vi "readString.vi"(8 "error in (no error)":errorcluster, 10 "Length":i32, 11 "ModbusBuffer in":refnum<class "ModbusBuffer.lvclass">) -> (0 "error out":errorcluster, 2 "Output":string, 3 "ModbusBuffer out":refnum<class "ModbusBuffer.lvclass">)   [LabVIEW 2016, in "RTModbus.lvlib" / "ModbusBuffer.lvclass"]
uses:
  ModbusBuffer.lvclass
  ModbusBuffer.lvclass/ModbusBuffer.ctl
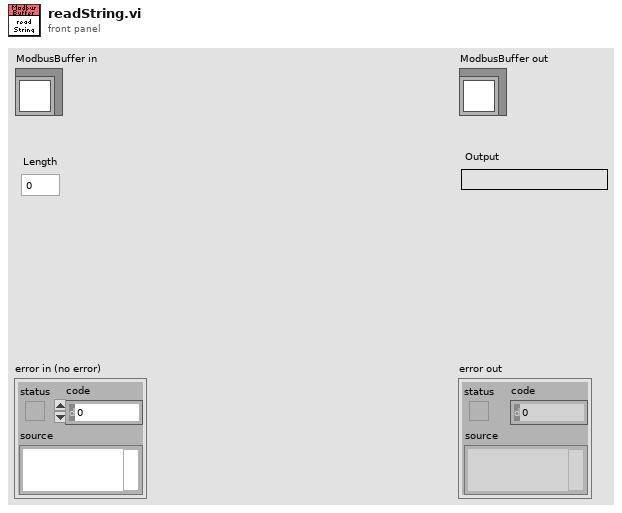
[diagram p1: front panel]
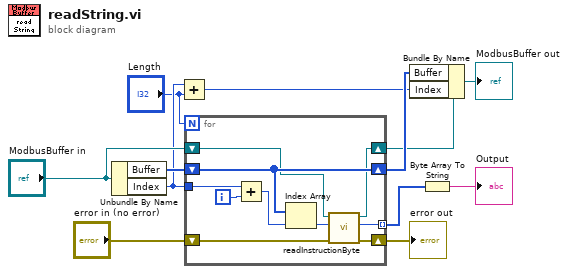
[diagram p0: block diagram]
diagram:
  n1 = Unbundle By Name("ModbusBuffer in") -> ("Buffer"=w11:u16[], "Index"=w5:i32)
  n2 = Add(x=w5, y="Length") -> (x+y=w3:i32)
  n3 = for {
    N: "Length" -> [_]
    tunnel: w5 -> [w15]
    shift-right: [w19] -> w7
    shift-left: "ModbusBuffer in" -> [w20]
    shift-right: [w22] -> w10
    shift-left: w11 -> [w22]
    shift-right: [w17] -> w8
    shift-left: "error in (no error)" -> [w18]
    tunnel: [w13] -> w2 mode=indexing
    i -> [w16]
    n4 = Add(x=w15, y=w16) -> (x+y=w14:i32)
    n5 = Index Array(array=w22, index=w14) -> (element=w21:u16)
    n6 = call "readInstructionByte.vi"("error in (no error)"=w18, "Instruction"=w21, "ModbusBuffer in"=w20) -> ("error out"=w17:errorcluster, "Output"=w13:u8, "ModbusBuffer out"=w19:refnum<class "ModbusBuffer.lvclass">)  [unwired: 6 in]
  }
  "error out" <- w8
  n7 = Bundle By Name(cluster=w7, "Buffer"=w10, "Index"=w3) -> (→"ModbusBuffer out":refnum<class "ModbusBuffer.lvclass">)
  n8 = Byte Array To String(unsigned byte array=w2) -> (string=→"Output":string)
